vi "Add Message.vi"(8 "error in":errorcluster, 9 "messageAddresses":T1[](array[typedef]) {"direction" items=["Rx", "Tx"]}, 10 "message configuration":T2 {"messageType" items=["BCtoRT", "RTtoBC", "RTtoRT", "MC"]}, 11 "channel in":refnum<k24>) -> (0 "error out":errorcluster, 2 "new message":refnum<k24>, 3 "channel out":refnum<k24>)   [LabVIEW 2020, in "AIM_1553_Parameter_ni.lvlib"]
uses:
  AIM_1553_Parameter_ni.lvlib
  C:/Users/Administrator/Desktop/GIT/Ballard-Arinc-429-XML-Generator/Source/Assemblies/Aim_1553_Parameter_ni/bin/Debug/AIM_1553_Parameter_ni.dll
  Assemblies/Aim_1553_Parameter_ni/bin/Debug/AIM_1553_Parameter_ni.dll
  _tyedefs/message_type.ctl
  _tyedefs/messageAddress_type.ctl
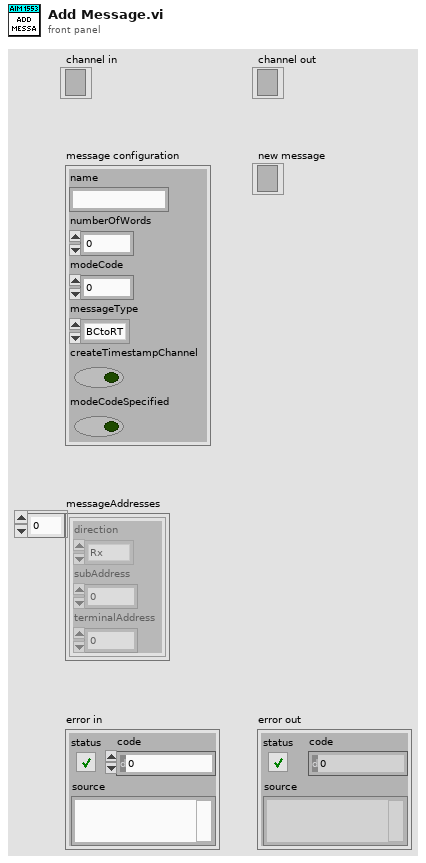
[diagram p1: front panel]
types:
  T1 = typedef "AIM_1553_Parameter_ni.lvlib/messageAddress_type.ctl" = cluster{"direction":i32, "subAddress":i32, "terminalAddress":i32}
  T2 = typedef "AIM_1553_Parameter_ni.lvlib/message_type.ctl" = cluster{"name":string, "numberOfWords":i32, "modeCode":i32, "messageType":i32, "createTimestampChannel":bool, "modeCodeSpecified":bool}
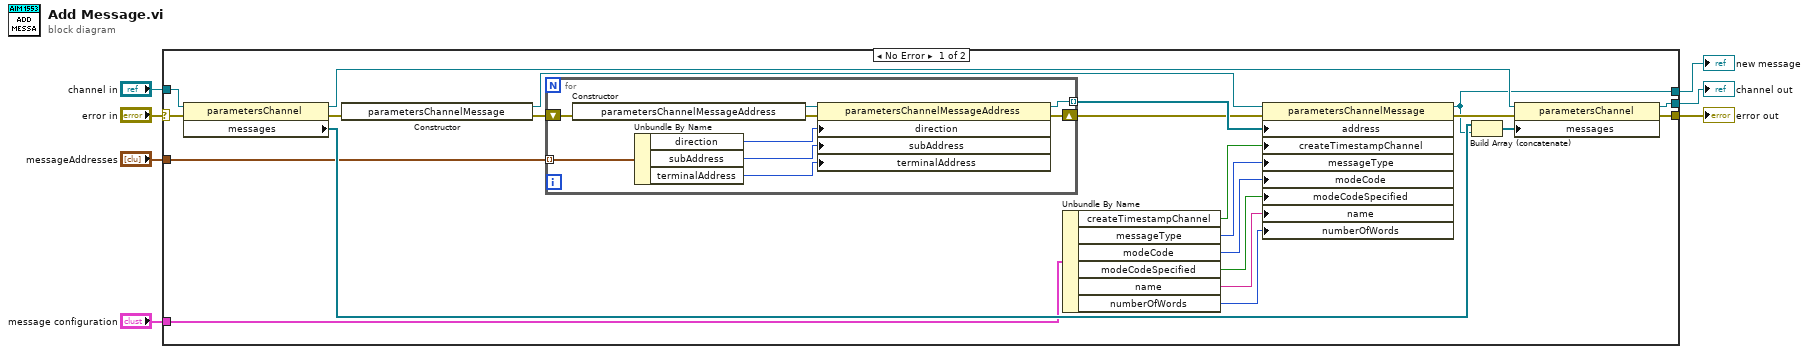
[diagram p0: block diagram]
diagram:
  n1 = case shown="No Error" "error in" {
    selector: "error in" -> [w28 w39]
    tunnel: [w26 w40] -> w7
    tunnel: [w25 w39] -> w6
    tunnel: "channel in" -> [w29 w40]
    tunnel: [w19 _] -> w3
    tunnel: "message configuration" -> [w18 _]
    tunnel: "messageAddresses" -> [w8 _]
    frame No Error {
      n2 = property class="parametersChannel"(reference=w29, error in=w28) -> (reference out=w27:refnum<k24>, error out=w22:errorcluster, "messages"=w23:refnum<k24>[])
      n3 = constructor class="parametersChannelMessage"(error in=w22) -> (reference out=w24:refnum<k24>, error out=w11:errorcluster)  [unwired: 2 in, 1 out]
      n4 = for {
        shift-right: [w35] -> w9
        shift-left: w11 -> [w36]
        tunnel: [w34] -> w10 mode=indexing
        tunnel: w8 -> [w33] mode=indexing
        n5 = constructor class="parametersChannelMessageAddress"(error in=w36) -> (reference out=w38:refnum<k24>, error out=w37:errorcluster)  [unwired: 2 in, 1 out]
        n6 = Unbundle By Name(w33) -> ("direction"=w32:i32, "subAddress"=w31:i32, "terminalAddress"=w30:i32)
        n7 = property class="parametersChannelMessageAddress"(reference=w38, error in=w37, "direction"=w32, "subAddress"=w31, "terminalAddress"=w30) -> (reference out=w34:refnum<k24>, error out=w35:errorcluster)
      }
      n8 = Unbundle By Name(w18) -> ("createTimestampChannel"=w12:bool, "messageType"=w13:i32, "modeCode"=w14:i32, "modeCodeSpecified"=w15:bool, "name"=w16:string, "numberOfWords"=w17:i32)
      n9 = property class="parametersChannelMessage"(reference=w24, error in=w9, "address"=w10, "createTimestampChannel"=w12, "messageType"=w13, "modeCode"=w14, "modeCodeSpecified"=w15, "name"=w16, "numberOfWords"=w17) -> (reference out=w19:refnum<k24>, error out=w21:errorcluster)
      n10 = Build Array (concatenate)(w23, w19) -> (w20:refnum<k24>[])
      n11 = property class="parametersChannel"(reference=w27, error in=w21, "messages"=w20) -> (reference out=w26:refnum<k24>, error out=w25:errorcluster)
    }
    frame Error {
    }
  }
  "channel out" <- w7
  "error out" <- w6
  "new message" <- w3
